vi "Terminate.vi"(8 "error in (no error)":errorcluster, 10 "Message in":refnum<class "TerminateMessage.lvclass">, 11 "Piezo in":refnum<class "Piezo.lvclass">) -> (0 "error out":errorcluster, 3 "Piezo out":refnum<class "Piezo.lvclass">)   [LabVIEW 2012, in "Piezo.lvclass"]
doc: "This member function is called when the statemachine in the run.vi receives an 'terminate' command. It closes the RabbitMQ connection. \n\nOverride this member function in your derived class to release all previously acquired resources (but don't forget to call the parent method). If your component has subcomponents, they count as resources, and you have to release them by calling their own terminate functions."
uses:
  Piezo.lvclass
  <vilib>/Distrio/Murmex/TerminateMessage/TerminateMessage.lvclass
  <vilib>/Distrio/Murmex/Murmex/Murmex.lvclass
  Piezo.lvclass/Piezo.ctl
panel:
  # "This method is called when the TERMINATE\ntrigger is sent. \n\nOverride this method when your component needs to\nrespond to this trigger. \n\nCall parent for proper implementation"
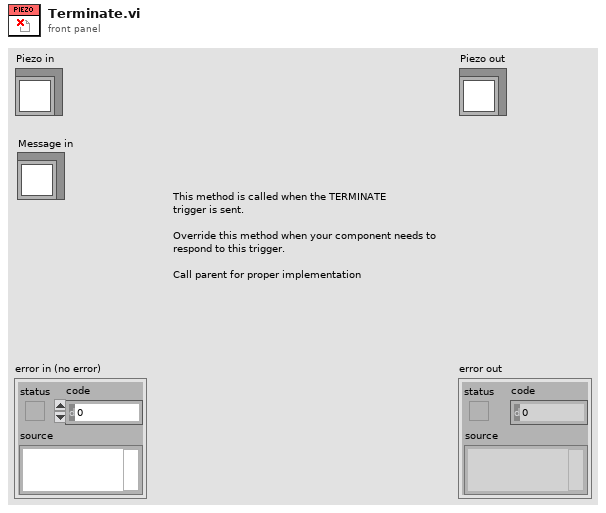
[diagram p1: front panel]
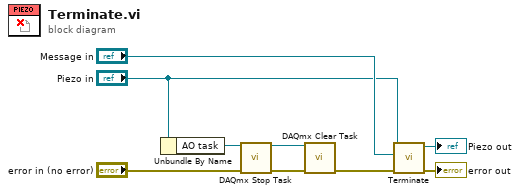
[diagram p0: block diagram]
diagram:
  n1 = Unbundle By Name("Piezo in") -> ("AO task"=w1:refnum<k21>)
  n2 = call <vilib>:"DAQmx Stop Task.vi"("task/channels in"=w1, "error in"="error in (no error)") -> ("task out"=w5:refnum<k21>, "error out"=w4:errorcluster)  [unwired: 12 in]
  n3 = call <vilib>:"DAQmx Clear Task.vi"("task in"=w5, "error in"=w4) -> ("error out"=w2:errorcluster)  [unwired: 13 in]
  n4 = call-parent "Terminate.vi"("error in (no error)"=w2, "Message in"="Message in", "Murmex in"="Piezo in") -> ("error out"=→"error out":errorcluster, "Murmex out"=→"Piezo out":refnum<class "Piezo.lvclass">)  [unwired: 7 in]
